vi "Configure Lan Trigger.vi"(5 "Enable Lan State (T: Enable)":bool=TRUE, 6 "IP Address (\"0.0.0.0\")":string="0.0.0.0", 7 "Logic Type (1: Negative)":i32(ring)=1 items=["Positive", "Negative"], 8 "error in (no error)":errorcluster, 9 "LAN Stimulus Event (\"NONE\")":string="NONE", 10 "LAN Number (1: Lan 1)":i32(ring)=1 items=["Lan 1"=1, "Lan 2"=2, "Lan 3"=3, "Lan 4"=4, "Lan 5"=5, "Lan 6"=6, "Lan 7"=7, "Lan 8"=8], 11 "VISA resource name":refnum<visa-resource-name>) -> (0 "error out":errorcluster, 3 "VISA resource name out":refnum<visa-resource-name>)   [LabVIEW 2015, in "Keithley DMM6500 DAQ6500 Series.lvlib"]
doc: "Prepares the event generator for outgoing trigger events, specifies the address (in dotted-decimal format) of UDP or TCP listeners, sets the logic on which the trigger event detector and the output trigger generator operate on the given trigger line, sets the LAN protocol to use for sending trigger messages and specifies events that cause this trigger to assert."
uses:
  <instrlib>/Keithley DMM6500 DAQ6500 Series/Keithley DMM6500 DAQ6500 Series.lvlib
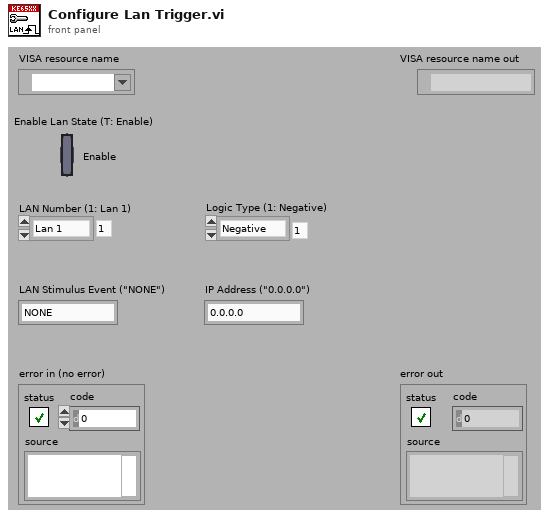
[diagram p1: front panel]
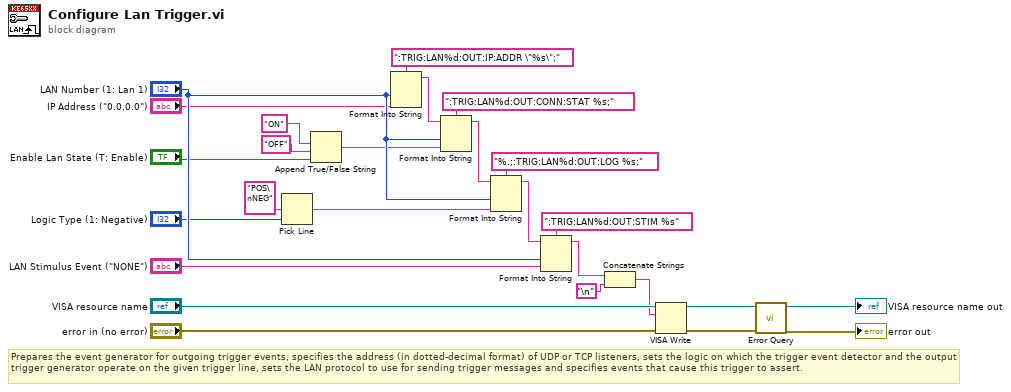
[diagram p0: block diagram]
diagram:
  # "Prepares the event generator for outgoing trigger events, specifies the address (in dotted-decimal format) of UDP or TCP listeners, sets the logic on which the trigger event detector and the output trigger generator operate on the given trigger line, sets the LAN protocol to use for sending trigger messages and specifies events that cause this trigger to assert."
  n1 = Pick Line(multi-line string="POS\nNEG", line index="Logic Type (1: Negative)") -> (output string=w4:string)  [unwired: 1 in]
  n2 = Append True/False String(1:"Enable Lan State (T: Enable)", 2:"OFF", 3:"ON") -> (0:w18:string)  [unwired: 1 in]
  n3 = Format Into String(format string=":TRIG:LAN%d:OUT:IP:ADDR \"%s\";", "LAN Number (1: Lan 1)", "IP Address (\"0.0.0.0\")") -> (resulting string=w20:string)  [unwired: 2 in, 1 out]
  n4 = Format Into String(format string=":TRIG:LAN%d:OUT:CONN:STAT %s;", initial string=w20, "LAN Number (1: Lan 1)", w18) -> (resulting string=w17:string)  [unwired: 1 in, 1 out]
  n5 = Format Into String(format string="%.;:TRIG:LAN%d:OUT:LOG %s;", initial string=w17, "LAN Number (1: Lan 1)", w4) -> (resulting string=w15:string)  [unwired: 1 in, 1 out]
  n6 = Format Into String(format string=":TRIG:LAN%d:OUT:STIM %s", initial string=w15, "LAN Number (1: Lan 1)", "LAN Stimulus Event (\"NONE\")") -> (resulting string=w2:string)  [unwired: 1 in, 1 out]
  n7 = Concatenate Strings(w2, "\n") -> (w3:string)
  n8 = VISA Write(VISA resource name="VISA resource name", write buffer=w3, error in (no error)="error in (no error)") -> (VISA resource name out=w10:refnum<visa-resource-name>, error out=w9:errorcluster)  [unwired: 1 out]
  n9 = call <instrlib>:"Error Query.vi"("error in (no error)"=w9, "VISA resource name"=w10) -> ("error out"=→"error out":errorcluster, "VISA resource name out"=→"VISA resource name out":refnum<visa-resource-name>)  [unwired: 6 in, 2 out]
